vi "ke37xx Configure Channel Matching.vi"(0 "VISA Resource Name":refnum<visa-resource-name>, 1 "Width (1)":u8=1, 2 "Match State Latching (True)":bool, 5 "Specified Channels":string, 7 "Match Value":u32, 9 "Matching Type (0:Exact)":T1(ring), 11 "error in (no error)":errorcluster, 12 "Channel Mask":string) -> (4 "VISA Resource Name Out":refnum<visa-resource-name>, 15 "error out":errorcluster)   [LabVIEW 2009, in "Keithley 3700 Series.lvlib"]
doc: "This VI configures a channel for matching a specified value. Used on Totalizer and Digital I/O channels."
uses:
  <instrlib>/Keithley 3706/Keithley 3700 Series.lvlib
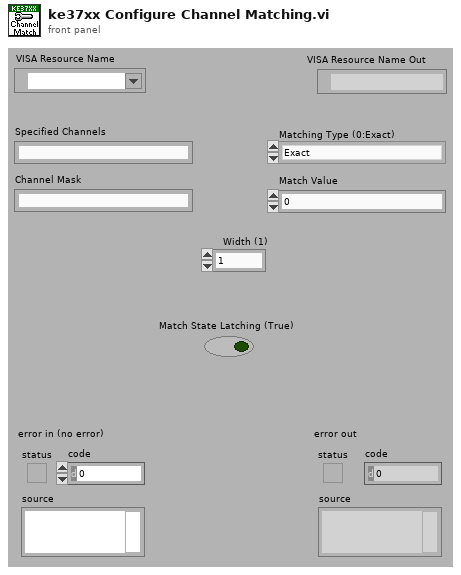
[diagram p1: front panel]
types:
  T1 = enum16{"Exact", "Match Any", "Match Not Exact", "None"}
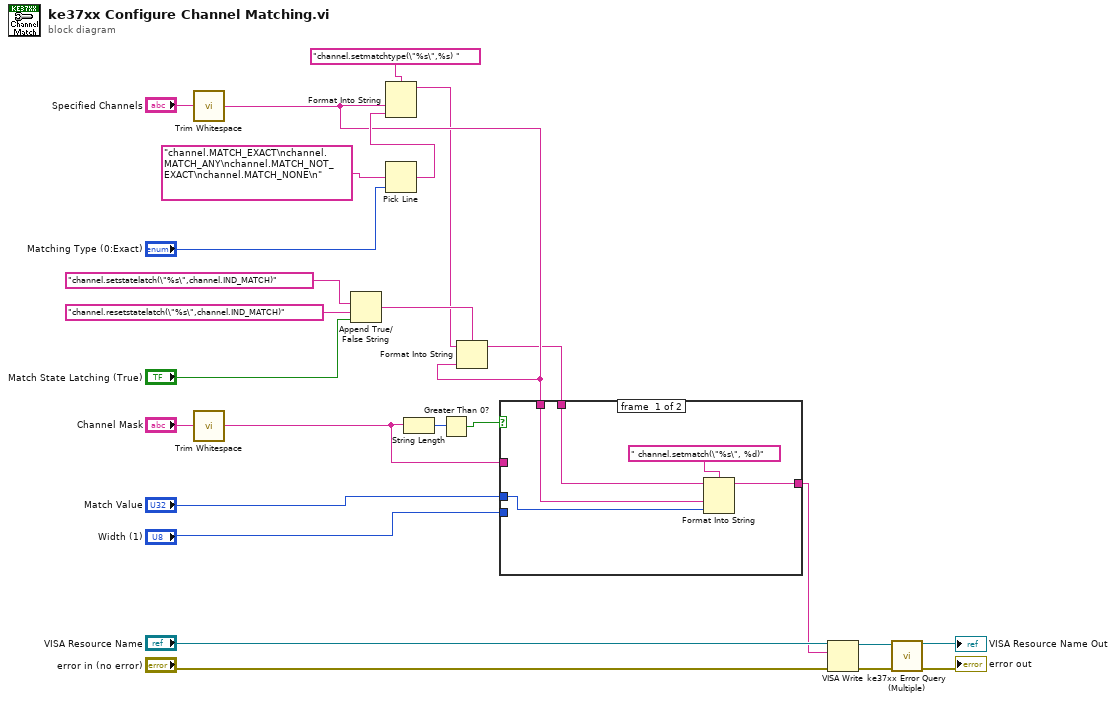
[diagram p0: block diagram]
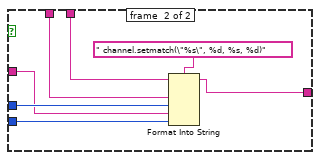
[diagram p2: hidden frame]
diagram:
  n1 = call <vilib>:"Trim Whitespace.vi"("string"="Specified Channels") -> ("trimmed string"=w5:string)  [unwired: 1 in]
  n2 = call <vilib>:"Trim Whitespace.vi"("string"="Channel Mask") -> ("trimmed string"=w11:string)  [unwired: 1 in]
  n3 = Append True/False String(1:"Match State Latching (True)", 2:"channel.resetstatelatch(\"%s\",channel.IND_MATCH)", 3:"channel.setstatelatch(\"%s\",channel.IND_MATCH)") -> (0:w6:string)  [unwired: 1 out]
  n4 = Pick Line(multi-line string="channel.MATCH_EXACT\nchannel.MATCH_ANY\nchannel.MATCH_NOT_EXACT\nchannel.MATCH_NONE\n", line index="Matching Type (0:Exact)") -> (output string=w16:string)  [unwired: 1 out]
  n5 = Format Into String(format string="channel.setmatchtype(\"%s\",%s) ", w5, w16) -> (resulting string=w4:string)  [unwired: 2 in, 1 out]
  n6 = String Length(string=w11) -> (length=w15:i32)
  n7 = Greater Than 0?(x=w15) -> (x > 0?=w14:bool)
  n8 = Format Into String(format string=w6, initial string=w4, w5) -> (resulting string=w3:string)  [unwired: 1 in, 1 out]
  n9 = case shown="True" w14 {
    tunnel: w3 -> [w28 w36]
    tunnel: "Match Value" -> [w27 w35]
    tunnel: w11 -> [_ w34]
    tunnel: "Width (1)" -> [_ w33]
    tunnel: w5 -> [w29 w32]
    tunnel: [w26 w31] -> w13
    frame #0 {
      n10 = Format Into String(format string=" channel.setmatch(\"%s\", %d)", initial string=w28, w29, w27) -> (resulting string=w26:string)  [unwired: 1 in, 1 out]
    }
    frame #1 {
      n11 = Format Into String(format string=" channel.setmatch(\"%s\", %d, %s, %d)", initial string=w36, w32, w35, w34, w33) -> (resulting string=w31:string)  [unwired: 1 in, 1 out]
    }
  }
  n12 = VISA Write(VISA resource name="VISA Resource Name", write buffer=w13, error in (no error)="error in (no error)") -> (VISA resource name out=w20:refnum<visa-resource-name>, error out=w19:errorcluster)  [unwired: 1 out]
  n13 = call <instrlib>:"ke37xx Error Query (Multiple).vi"("VISA resource name"=w20, "error in (no error)"=w19) -> ("VISA resource name out"=→"VISA Resource Name Out":refnum<visa-resource-name>, "error out"=→"error out":errorcluster)  [unwired: 12 out]
